vi "Layout.vi"(8 "Error In":errorcluster, 11 "reference in":refnum<class "DemoApplication.lvclass">) -> (0 "Error Out":errorcluster, 3 "reference in":refnum<class "DemoApplication.lvclass">)   [LabVIEW 2021, in "DemoApplication.lvclass"]
uses:
  DemoApplication.lvclass
  c12fd466-6d7f-429f-8d31-7d2924c23ef2.vi
  <vilib>/Utility/Data Type/Get Cluster Information.vi
  <vilib>/Utility/Data Type/Get Type Information.vi
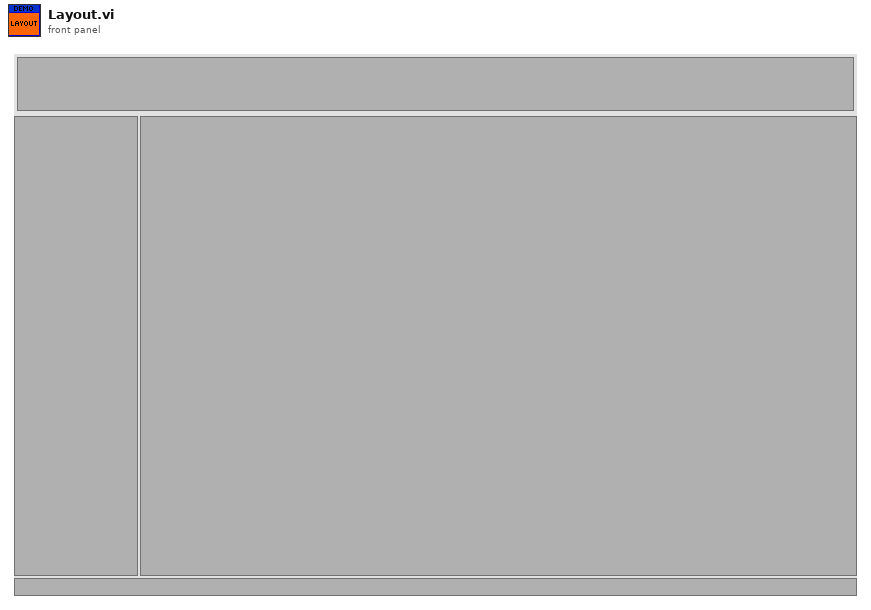
[diagram p1: front panel]
types:
  T1 = cluster{"Header":refnum<vi>, "ButtonBar":refnum<vi>, "MainFlexPanel":refnum<vi>, "Footer":refnum<vi>}
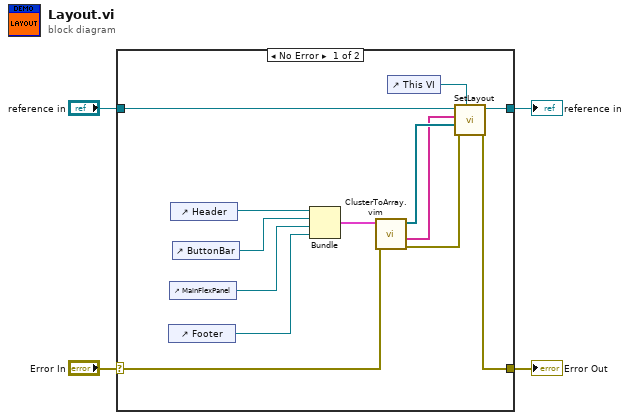
[diagram p0: block diagram]
diagram:
  n1 = case shown="No Error" "Error In" {
    selector: "Error In" -> [w12 w19]
    tunnel: [w5 w19] -> w3
    tunnel: [w11 w18] -> w1
    tunnel: "reference in" -> [w10 w18]
    frame No Error {
      n2 = control-ref of="Footer"() -> (w16:refnum<vi>)
      n3 = control-ref of="MainFlexPanel"() -> (w15:refnum<vi>)
      n4 = control-ref of="Header"() -> (w13:refnum<vi>)
      n5 = control-ref of="ButtonBar"() -> (w14:refnum<vi>)
      n6 = Bundle("Header"=w13, "ButtonBar"=w14, "MainFlexPanel"=w15, "Footer"=w16) -> (w17:T1)  [unwired: 1 in]
      n7 = call "ClusterToArray.vim"("Error In"=w12, "Cluster"=w17) -> ("Error Out"=w6:errorcluster, "Labels"=w7:string[], "ArrayOfElements"=w8:refnum<vi>[])  [unwired: 7 in]
      n8 = control-ref of="This VI"() -> (w9:refnum<vi>)
      n9 = call-dynamic "SetLayout.vi"("PanelVIRef"=w9, "Error In"=w6, "SubPanels"=w8, "Labels"=w7, "reference in"=w10) -> ("Error Out"=w5:errorcluster, "reference in"=w11:refnum<class "DemoApplication.lvclass">)  [unwired: 5 in]
    }
    frame Error {
    }
  }
  "Error Out" <- w3
  "reference in" <- w1
